vi "AlliGator Get Gate Indices to Load.vi"(4 "Gates to?":bool, 6 "Gates to Use":T1, 8 "Error In":errorcluster, 9 "Gate Step":i32, 11 "Gate Indices in":i32[](array[numeric])) -> (0 "Error Out":errorcluster, 1 "Gates across boundaries?":bool, 2 "Split Index":u32, 3 "Gate Indices out":i32[](array[numeric]))   [LabVIEW 2021, in "AlliGator Files.lvlib"]
doc: "Gets the gate indices to load."
uses:
  AlliGator Files.lvlib
  Settings/AlliGator Background Subtraction Parameters.ctl
  7d0e7d68-c0d6-4156-aa84-201d3fec3c70.vi
  Settings/AlliGator Settings.lvlib
panel:
  # "see the AlliGator License on the block diagram (Ctrl+E or Window:Show Block Diagram)"
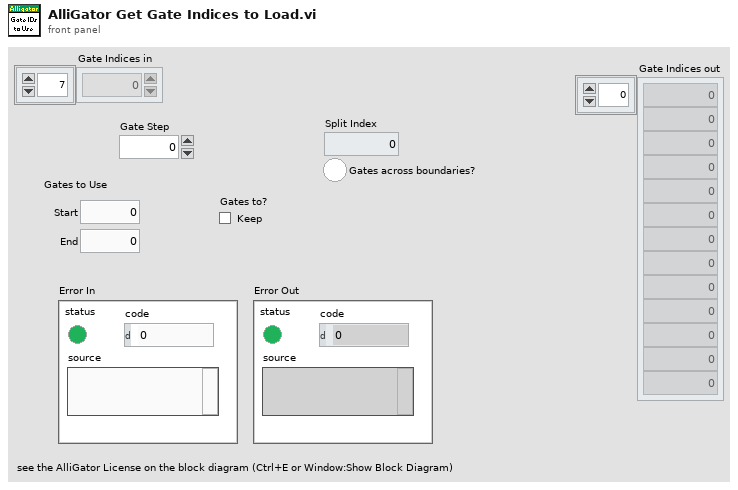
[diagram p1: front panel]
types:
  T1 = typedef "AlliGator Settings.lvlib/AlliGator Background Subtraction Parameters.ctl" = cluster{"Start":u32, "End":u32}
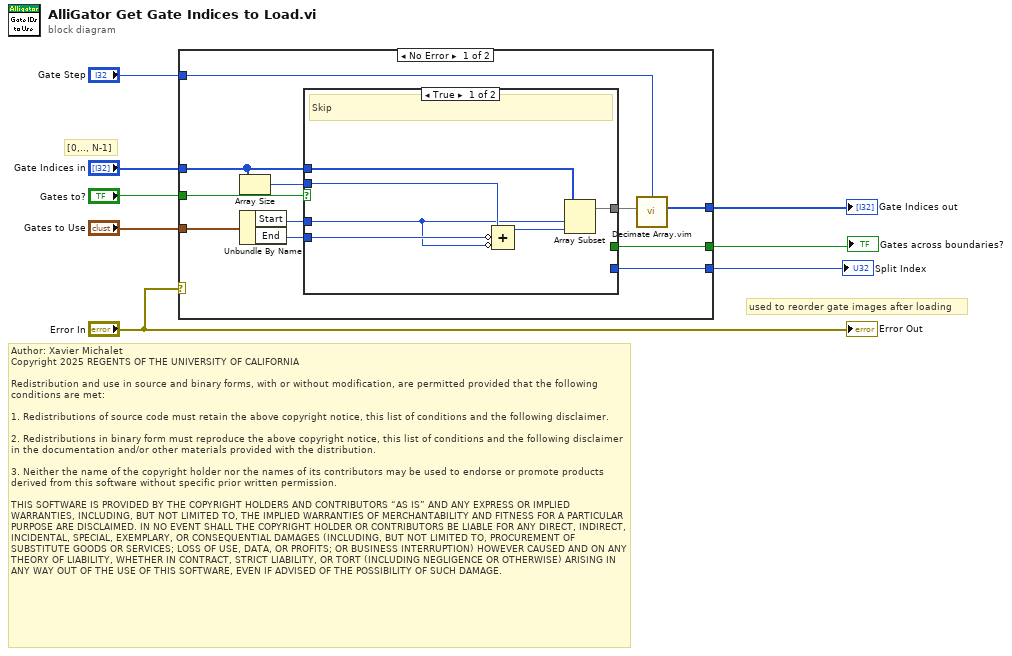
[diagram p0: block diagram]
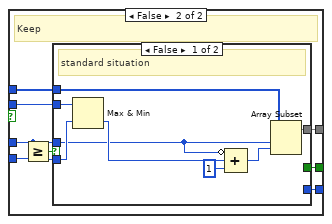
[diagram p2: hidden frame]
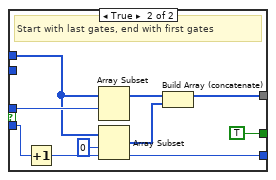
[diagram p3: hidden frame]
diagram:
  # "Author: Xavier Michalet\nCopyright 2025 REGENTS OF THE UNIVERSITY OF CALIFORNIA\n\nRedistribution and use in source and binary forms, with or without modification, are permitted provided that the following conditions are met:\n\n1. Redistributions of source code must retain the above copyright notice, this list of conditions and the following disclaimer.\n\n2. Redistributions in binary form must reproduce the above copyright notice, this list of conditions and the following disclaimer in the documentation and/or other materials provided with the distribution.\n\n3. Neither the name of the copyright holder nor the names of its contributors may be used to endorse or promote products derived from this software without specific prior written permission.\n\nTHIS SOFTWARE IS PROVIDED BY THE COPYRIGHT HOLDERS AND CONTRIBUTORS “AS IS” AND ANY EXPRESS OR IMPLIED WARRANTIES, INCLUDING, BUT NOT LIMITED TO, THE IMPLIED WARRANTIES OF MERCHANTABILITY AND FITNESS FOR A PARTICULAR PURPOSE ARE DISCLAIMED. IN NO EVENT SHALL THE COPYRIGHT HOLDER OR CONTRIBUTORS BE LIABLE FOR ANY DIRECT, INDIRECT, INCIDENTAL, SPECIAL, EXEMPLARY, OR CONSEQUENTIAL DAMAGES (INCLUDING, BUT NOT LIMITED TO, PROCUREMENT OF SUBSTITUTE GOODS OR SERVICES; LOSS OF USE, DATA, OR PROFITS; OR BUSINESS INTERRUPTION) HOWEVER CAUSED AND ON ANY THEORY OF LIABILITY, WHETHER IN CONTRACT, STRICT LIABILITY, OR TORT (INCLUDING NEGLIGENCE OR OTHERWISE) ARISING IN ANY WAY OUT OF THE USE OF THIS SOFTWARE, EVEN IF ADVISED OF THE POSSIBILITY OF SUCH DAMAGE."
  # "used to reorder gate images after loading"
  # "[0,.., N-1]"
  n1 = case shown="No Error" "Error In" {
    tunnel: "Gate Step" -> [w19 _]
    tunnel: "Gates to Use" -> [w18 _]
    tunnel: [w17 w51] -> w6
    tunnel: "Gates to?" -> [w15 _]
    tunnel: "Gate Indices in" -> [w14 w51]
    tunnel: [w10 _] -> w3
    tunnel: [w9 _] -> w2
    frame No Error {
      n2 = Array Size(array=w14) -> (size(s)=w13:i32)
      n3 = Unbundle By Name(w18) -> ("Start"=w12:u32, "End"=w11:u32)
      n4 = case shown="True" w15 {
        tunnel: [w25 w33] -> w16
        tunnel: w14 -> [w23 w32]
        tunnel: w13 -> [w22 w31]
        tunnel: w11 -> [w21 w30]
        tunnel: w12 -> [w20 w29]
        tunnel: [_ w27] -> w10
        tunnel: [_ w26] -> w9
        frame True {
          # "Skip"
          n5 = Compound Arithmetic op=ADD(w22, invert w21, invert w20) -> (w24:u32)
          n6 = Array Subset(array=w23, index=w20, length=w24) -> (w25:i32[])
        }
        frame False {
          # "Keep"
          n7 = Greater Or Equal?(x=w29, y=w30) -> (x >= y?=w28:bool)
          n8 = case shown="False" w28 {
            tunnel: [w41 w45] -> w33
            tunnel: w32 -> [w40 w47]
            tunnel: w31 -> [w38 _]
            tunnel: w30 -> [w35 w48]
            tunnel: w29 -> [w34 w49]
            tunnel: [_ TRUE ("Gates across boundaries?")] -> w27
            tunnel: [_ w42] -> w26
            frame False {
              # "standard situation"
              n9 = Max & Min(x=w38, y=w35) -> (min(x,y)=w37:u32)  [unwired: 1 out]
              n10 = Compound Arithmetic op=ADD(invert w34, w37, u32 1 ("value")) -> (w39:u32)
              n11 = Array Subset(array=w40, index=w34, length=w39) -> (w41:i32[])
            }
            frame True {
              # "Start with last gates, end with first gates"
              n12 = Increment(x=w48) -> (x+1=w42:u32)
              n13 = Array Subset(array=w47, index=w49) -> (w50:i32[])  [unwired: 1 in]
              n14 = Array Subset(array=w47, index=0, length=w42) -> (w44:i32[])
              n15 = Build Array (concatenate)(w50, w44) -> (w45:i32[])
            }
          }
        }
      }
      n16 = call "Decimate Array.vim"("Decimation (1)"=w19, "Input Array"=w16) -> ("Decimated Array"=w17:i32[])  [unwired: 5 in]
    }
    frame Error {
    }
  }
  "Gate Indices out" <- w6
  "Gates across boundaries?" <- w3
  "Split Index" <- w2
  "Error Out" <- "Error In"
